vi "Initialize device.vi"(2 "error in (no error)":errorcluster, 3 "handle":u32) -> (0 "error out":errorcluster, 1 "success":bool)   [LabVIEW 2013]
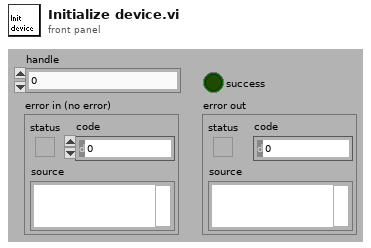
[diagram p1: front panel]
types:
  T1 = cluster{"ADBUS3ChipSelectPinState":bool, "ADBUS4GPIOL1PinState":bool, "ADBUS5GPIOL2PinState":bool, "ADBUS6GPIOL3PinState":bool, "ADBUS7GPIOL4PinState":bool}
  T2 = cluster{"Pin I/O State 1":bool, "Pin L/H State 1":bool, "Pin I/O State 2":bool, "Pin L/H State 2":bool, "Pin I/O State 3":bool, "Pin L/H State 3":bool, "Pin I/O State 4":bool, "Pin L/H State 4":bool, "Pin I/O State 5":bool, "Pin L/H State 5":bool, "Pin I/O State 6":bool, "Pin L/H State 6":bool, "Pin I/O State 7":bool, "Pin L/H State 7":bool, "Pin I/O State 8":bool, "Pin L/H State 8":bool}
  T3 = cluster{"Pin 1":bool, "Pin 2":bool, "Pin 3":bool, "Pin 4":bool, "Pin 5":bool, "Pin 6":bool, "Pin 7":bool, "Pin 8":bool}
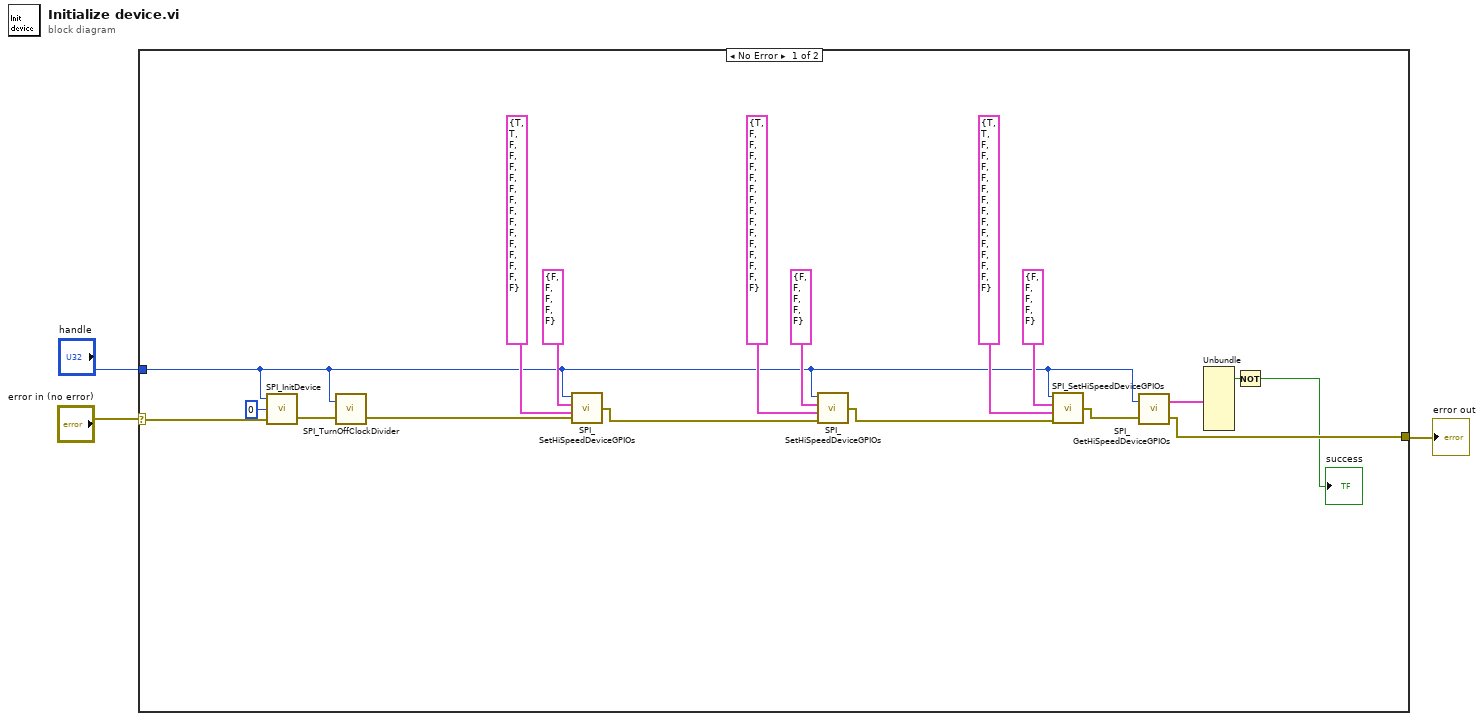
[diagram p0: block diagram]
diagram:
  n1 = case shown="No Error" "error in (no error)" {
    selector: "error in (no error)" -> [w8 w22]
    tunnel: [w13 w22] -> w3
    tunnel: "handle" -> [w4 _]
    frame No Error {
      n2 = call "SPI_InitDevice.vi"("error in (no error)"=w8, "clock divisor"=u32 0, "handle"=w4) -> ("error out"=w5:errorcluster)  [unwired: 2 out]
      n3 = call "SPI_TurnOffClockDivider.vi"("error in (no error)"=w5, "handle"=w4) -> ("error out"=w6:errorcluster)  [unwired: 1 out]
      n4 = call "SPI_SetHiSpeedDeviceGPIOs.vi"("error in (no error)"=w6, "high input output pins data"=T2 {"Pin I/O State 1"=TRUE, "Pin L/H State 1"=TRUE, "Pin I/O State 2"=FALSE, "Pin L/H State 2"=FALSE, "Pin I/O State 3"=FALSE, "Pin L/H State 3"=FALSE, "Pin I/O State 4"=FALSE, "Pin L/H State 4"=FALSE, "Pin I/O State 5"=FALSE, "Pin L/H State 5"=FALSE, "Pin I/O State 6"=FALSE, "Pin L/H State 6"=FALSE, "Pin I/O State 7"=FALSE, "Pin L/H State 7"=FALSE, "Pin I/O State 8"=FALSE, "Pin L/H State 8"=FALSE}, "chip selects disable states"=T1 {"ADBUS3ChipSelectPinState"=FALSE, "ADBUS4GPIOL1PinState"=FALSE, "ADBUS5GPIOL2PinState"=FALSE, "ADBUS6GPIOL3PinState"=FALSE, "ADBUS7GPIOL4PinState"=FALSE}, "handle"=w4) -> ("error out"=w11:errorcluster)
      n5 = call "SPI_SetHiSpeedDeviceGPIOs.vi"("error in (no error)"=w11, "high input output pins data"=T2 {"Pin I/O State 1"=TRUE, "Pin L/H State 1"=FALSE, "Pin I/O State 2"=FALSE, "Pin L/H State 2"=FALSE, "Pin I/O State 3"=FALSE, "Pin L/H State 3"=FALSE, "Pin I/O State 4"=FALSE, "Pin L/H State 4"=FALSE, "Pin I/O State 5"=FALSE, "Pin L/H State 5"=FALSE, "Pin I/O State 6"=FALSE, "Pin L/H State 6"=FALSE, "Pin I/O State 7"=FALSE, "Pin L/H State 7"=FALSE, "Pin I/O State 8"=FALSE, "Pin L/H State 8"=FALSE}, "chip selects disable states"=T1 {"ADBUS3ChipSelectPinState"=FALSE, "ADBUS4GPIOL1PinState"=FALSE, "ADBUS5GPIOL2PinState"=FALSE, "ADBUS6GPIOL3PinState"=FALSE, "ADBUS7GPIOL4PinState"=FALSE}, "handle"=w4) -> ("error out"=w15:errorcluster)
      n6 = call "SPI_SetHiSpeedDeviceGPIOs.vi"("error in (no error)"=w15, "high input output pins data"=T2 {"Pin I/O State 1"=TRUE, "Pin L/H State 1"=TRUE, "Pin I/O State 2"=FALSE, "Pin L/H State 2"=FALSE, "Pin I/O State 3"=FALSE, "Pin L/H State 3"=FALSE, "Pin I/O State 4"=FALSE, "Pin L/H State 4"=FALSE, "Pin I/O State 5"=FALSE, "Pin L/H State 5"=FALSE, "Pin I/O State 6"=FALSE, "Pin L/H State 6"=FALSE, "Pin I/O State 7"=FALSE, "Pin L/H State 7"=FALSE, "Pin I/O State 8"=FALSE, "Pin L/H State 8"=FALSE}, "chip selects disable states"=T1 {"ADBUS3ChipSelectPinState"=FALSE, "ADBUS4GPIOL1PinState"=FALSE, "ADBUS5GPIOL2PinState"=FALSE, "ADBUS6GPIOL3PinState"=FALSE, "ADBUS7GPIOL4PinState"=FALSE}, "handle"=w4) -> ("error out"=w14:errorcluster)
      n7 = call "SPI_GetHiSpeedDeviceGPIOs.vi"("error in (no error)"=w14, "handle"=w4) -> ("error out"=w13:errorcluster, "high pins input data"=w12:T3)
      n8 = Unbundle(w12) -> ("Pin 2"=w10:bool)  [unwired: 7 out]
      n9 = Not(x=w10) -> (.not. x?=→"success":bool)
    }
    frame Error {
    }
  }
  "error out" <- w3
